vi "PCT Init.vi"(11 "VI in":refnum<vi>) -> (0 "error out":errorcluster, 1 "Data REF":T2, 2 "Message Queues out":T1, 3 "User Event out":refnum<user-event>, 5 "Event Registration Refnum":refnum<event-registration>)   [LabVIEW 2020]
uses:
  PCT Data REFs.ctl
  <instrlib>/PalmSens SDK for LabVIEW 5.10/PalmSens/MeasurementResults.ctl
  <instrlib>/PalmSens SDK for LabVIEW 5.10/PalmSens/LiveCurveResult.ctl
  Message Queue/All Message Queues.ctl
  Message Queue/Message Cluster.ctl
  PCT FGV CMD.ctl
  User Event - Stop/User Event - Stop.lvlib
  Message Queue/Message Queue.lvlib
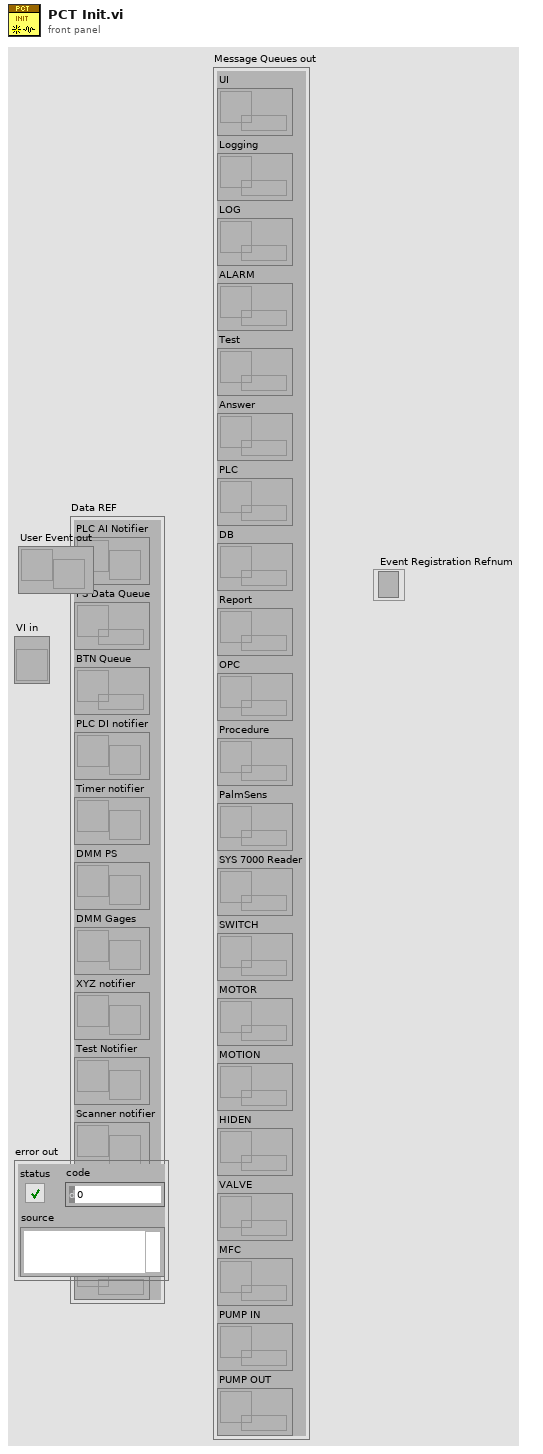
[diagram p1: front panel]
types:
  T1 = typedef "Message Queue.lvlib/All Message Queues.ctl" = cluster{"UI":refnum<queue>, "Logging":refnum<queue>, "LOG":refnum<queue>, "ALARM":refnum<queue>, "Test":refnum<queue>, "Answer":refnum<queue>, "PLC":refnum<queue>, "DB":refnum<queue>, "Report":refnum<queue>, "OPC":refnum<queue>, "Procedure":refnum<queue>, "PalmSens":refnum<queue>, "SYS 7000 Reader":refnum<queue>, "SWITCH":refnum<queue>, "MOTOR":refnum<queue>, "MOTION":refnum<queue>, "HIDEN":refnum<queue>, "VALVE":refnum<queue>, "MFC":refnum<queue>, "PUMP IN":refnum<queue>, "PUMP OUT":refnum<queue>}
  T2 = typedef "PCT Data REFs.ctl" = cluster{"PLC AI Notifier":refnum<notifier>, "PS Data Queue":refnum<queue>, "BTN Queue":refnum<queue>, "PLC DI notifier":refnum<notifier>, "Timer notifier":refnum<notifier>, "DMM PS":refnum<notifier>, "DMM Gages":refnum<notifier>, "XYZ notifier":refnum<notifier>, "Test Notifier":refnum<notifier>, "Scanner notifier":refnum<notifier>, "OPC Notifier":refnum<notifier>, "HIDEN queue":refnum<queue>}
  T3 = typedef "PCT FGV CMD.ctl" = enum16{"INIT", "GET", "SET"}
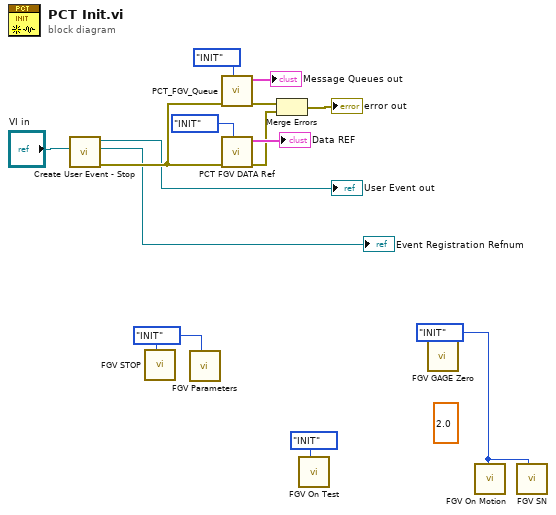
[diagram p0: block diagram]
diagram:
  (unwired) 2.0 ("input")
  w1 = PCT_FGV_CMD."INIT" ("CMD")
  w3 = PCT_FGV_CMD."INIT" ("CMD")
  n1 = call "Create User Event - Stop.vi"("VI in"="VI in") -> ("error out"=w13:errorcluster, "Event Registration Refnum"=→"Event Registration Refnum":refnum<event-registration>, "User Event"=→"User Event out":refnum<user-event>)  [unwired: 8 in]
  n2 = call "FGV STOP.vi"("CMD"=w3) -> ()  [unwired: 9 in, 2 out]
  n3 = call "FGV Parameters.vi"("CMD"=w3) -> ()  [unwired: 8 in, 3 out]
  n4 = call "PCT_FGV_Queue.vi"("CMD"=PCT_FGV_CMD."INIT", "error in (no error)"=w13) -> ("error out"=w9:errorcluster, "Message Queues out"=→"Message Queues out":T1)  [unwired: 8 in]
  n5 = call "PCT FGV DATA Ref.vi"("CMD"=PCT_FGV_CMD."INIT", "error in (no error)"=w13) -> ("error out"=w6:errorcluster, "Data REF"=→"Data REF":T2)  [unwired: 8 in]
  n6 = Merge Errors(w9, w6) -> (→"error out":errorcluster)
  n7 = call "FGV On Test.vi"("CMD"=PCT_FGV_CMD."INIT") -> ()  [unwired: 9 in, 2 out]
  n8 = call "FGV GAGE Zero.vi"("CMD"=w1) -> ()  [unwired: 9 in, 2 out]
  n9 = call "FGV On Motion.vi"("CMD"=w1) -> ()  [unwired: 9 in, 2 out]
  n10 = call "FGV SN.vi"("CMD"=w1) -> ()  [unwired: 9 in, 2 out]
